vi "reward_behavior_michelle_visjitter_conswinAdapt_enticefx_TSLog_VF_fortraining_lightdetection2.vi"() -> ()   [LabVIEW 2019]
doc: "The myRIO Project template acquires acceleration data from the onboard accelerometer and displays the changes of acceleration values in a waveform chart."
uses:
  <vilib>/Analysis/Matrix/Datatypes/RealMatrix.ctl
  <vilib>/myRIO/Instrument Drivers/Onboard IO/DIO/typedefs/DIO Reference.ctl
  <vilib>/myRIO/Common/Instrument Driver Framework/Utilities/typedefs/myRIO Generic Hardware Reference.ctl
  <vilib>/myRIO/Common/Instrument Driver Framework/Utilities/typedefs/Hardware Version Enum.ctl
  <vilib>/myRIO/Common/Instrument Driver Framework/Utilities/typedefs/myRIO v1.0 Reference.ctl
  <vilib>/myRIO/Common/Instrument Driver Framework/Utilities/typedefs/Generic FPGA Reference.ctl
  <vilib>/myRIO/Common/Instrument Driver Framework/myRIO v1.0/DIO/typedefs/DIO Channels List.ctl
  <vilib>/myRIO/Common/Instrument Driver Framework/myRIO v1.0/DIO/typedefs/DIO Channels Enum.ctl
  <vilib>/userdefined/High Color/nirio_resource_hc.ctl
  <vilib>/myRIO/Common/Instrument Driver Framework/myRIO v1.0/Encoder/typedefs/Encoder Signal Mode.ctl
  <vilib>/myRIO/Instrument Drivers/Onboard IO/Encoder/typedefs/Encoder Reference.ctl
  <vilib>/myRIO/Common/Instrument Driver Framework/myRIO v1.0/Encoder/typedefs/Encoder Channels Enum.ctl
  <vilib>/myRIO/Common/Instrument Driver Framework/myRIO v1.0/Encoder/typedefs/Encoder Configuration v1.0.ctl
  <vilib>/myRIO/Instrument Drivers/Onboard IO/AI/typedefs/AI Reference.ctl
  <vilib>/myRIO/Common/Instrument Driver Framework/myRIO v1.0/AI/typedefs/AI Channels List.ctl
  <vilib>/myRIO/Common/Instrument Driver Framework/myRIO v1.0/AI/typedefs/AI Channels Enum.ctl
  <vilib>/myRIO/Common/Instrument Driver Framework/Utilities/typedefs/Analog Scaling Constants List.ctl
  <vilib>/myRIO/Common/Instrument Driver Framework/Utilities/typedefs/Analog Scaling Constants.ctl
  <vilib>/myRIO/Common/Instrument Driver Framework/Utilities/vis/Is FPGA Ref Available.vi
  <vilib>/myRIO/Common/Instrument Driver Framework/myRIO v1.0/DIO/vis/myRIO v1.1 Open DIO.vi
  <vilib>/myRIO/Instrument Drivers/Onboard IO/DIO/vis/Write.vi
  <vilib>/myRIO/Common/Instrument Driver Framework/myRIO v1.0/Encoder/vis/myRIO v1.1 Open Encoder.vi
  <vilib>/myRIO/Instrument Drivers/Onboard IO/Encoder/vis/Read.vi
  <vilib>/myRIO/Common/Instrument Driver Framework/myRIO v1.0/AI/vis/myRIO v1.1 Open AI.vi
  <vilib>/myRIO/Instrument Drivers/Onboard IO/AI/vis/Read.vi
  <vilib>/myRIO/Instrument Drivers/Onboard IO/DIO/vis/Read.vi
  <vilib>/myRIO/Common/Instrument Driver Framework/Utilities/vis/Validate Channels.vi
  <vilib>/myRIO/Common/Instrument Driver Framework/myRIO v1.0/DIO/vis/myRIO v1.0 Reserve DIO.vi
  <vilib>/myRIO/Common/Instrument Driver Framework/myRIO v1.0/Encoder/vis/myRIO v1.0 Reserve Encoder.vi
  <vilib>/myRIO/Common/Instrument Driver Framework/myRIO v1.0/AI/vis/myRIO v1.0 Reserve AI.vi
  <vilib>/myRIO/Common/Instrument Driver Framework/myRIO v1.0/Resource Manager/vis/myRIO v1.0 Reserve Channel List.vi
  <vilib>/myRIO/Common/Instrument Driver Framework/myRIO v1.0/DIO/vis/myRIO v1.0 Build MUX Configuration DIO.vi
  <vilib>/myRIO/Common/Instrument Driver Framework/myRIO v1.0/Encoder/vis/myRIO v1.0 Build MUX Configuration Encoder.vi
  <vilib>/myRIO/Common/Instrument Driver Framework/myRIO v1.0/AI/vis/myRIO v1.0 Build MUX Configuration AI.vi
  <vilib>/myRIO/Common/Instrument Driver Framework/myRIO v1.0/Resource Manager/vis/myRIO v1.0 Reserve Channel.vi
  <vilib>/myRIO/Common/Instrument Driver Framework/myRIO v1.0/Resource Manager/vis/myRIO v1.0 Unreserve Channel.vi
  <vilib>/myRIO/Common/Instrument Driver Framework/myRIO v1.0/Resource Manager/vis/myRIO v1.0 Create Configuration List.vi
  <vilib>/myRIO/Common/Instrument Driver Framework/myRIO v1.0/Resource Manager/vis/myRIO v1.0 Build Mutex Name.vi
  <vilib>/Utility/VariantDataType/GetNumericInfo.vi
  <vilib>/Utility/error.llb/Error Cluster From Error Code.vi
  <vilib>/myRIO/Common/Instrument Driver Framework/myRIO v1.0/myRIO v1.1 Open.vi
  <vilib>/myRIO/Common/Instrument Driver Framework/Utilities/vis/IO Manager.vi
  <vilib>/myRIO/Common/Instrument Driver Framework/Utilities/vis/Configuration Manager.vi
  <vilib>/myRIO/Common/Instrument Driver Framework/myRIO v1.0/Resource Manager/vis/myRIO v1.0 Configure IO.vi
  <vilib>/myRIO/Common/Instrument Driver Framework/myRIO v1.0/myRIO v1.0 Close.vi
  <vilib>/myRIO/Common/Instrument Driver Framework/myRIO v1.0/Encoder/vis/myRIO v1.0 Configure Encoder.vi
  <vilib>/myRIO/Common/Instrument Driver Framework/myRIO v1.0/Encoder/vis/myRIO v1.0 Read Encoder.vi
  <vilib>/myRIO/Common/Instrument Driver Framework/myRIO v1.0/DIO/vis/myRIO v1.0 Write DIO.vi
  <vilib>/myRIO/Common/Instrument Driver Framework/myRIO v1.0/DIO/vis/myRIO v1.0 Read DIO.vi
  <vilib>/myRIO/Common/Instrument Driver Framework/myRIO v1.0/AI/vis/myRIO v1.0 Get Scaling Constants AI.vi
  <vilib>/myRIO/Common/Instrument Driver Framework/myRIO v1.0/AI/vis/myRIO v1.0 Read AI.vi
  <vilib>/myRIO/Express VI/Onboard IO/Encoder/Encoder Express VI.xnode
  <vilib>/myRIO/Instrument Drivers/Onboard IO/Encoder/vis/myRIO Encoder Open.xnode
  <vilib>/myRIO/Common/Instrument Driver Framework/myRIO v1.0/Encoder/typedefs/Encoder Count Direction Enum.ctl
  <vilib>/myRIO/Express VI/Onboard IO/DO/DO Express VI.xnode
  <vilib>/myRIO/Instrument Drivers/Onboard IO/DIO/vis/myRIO DIO Open.xnode
  <vilib>/myRIO/Express VI/Onboard IO/DI/DI Express VI.xnode
  <vilib>/myRIO/Express VI/Onboard IO/AI/AI Express VI.xnode
  <vilib>/myRIO/Instrument Drivers/Onboard IO/AI/vis/myRIO AI Open.xnode
  <vilib>/myRIO/Instrument Drivers/Onboard IO/Encoder/Encoder.lvlib
  <vilib>/myRIO/Instrument Drivers/Onboard IO/DIO/DIO.lvlib
  <vilib>/myRIO/Instrument Drivers/Onboard IO/AI/AI.lvlib
  <vilib>/Analysis/Matrix/NI_Matrix.lvlib
panel:
  out "LightDeriv":dbl
  out "LightOn":bool=TRUE
  out "Light":dbl
  out "Lightplot":dbl[](graph)
  out "LightArray":dbl[](array[numeric])
  out "AutoEnticeLimit":i32=1000
  out "GetVidFrame":i32
  out "VidTS":dbl[][](array[numeric])
  out "VidFrameClock":i32
  out "EntTS":dbl[][](array[numeric])
  out "TimeLag":dbl
  out "Lag2":dbl
  out "TestTime":dbl
  out "RewTS":dbl[][](array[numeric])
  out "ConsTS":dbl[][](array[numeric])
  out "LickTS":dbl[][](array[numeric])
  out "ContrastChoice":dbl
  out "Its":i32
  out "BurstCriteria":dbl
  out "LickBurst 2":bool
  out "LickBurst":bool
  out "Enticements":i32
  in  "Entice":bool
  out "Misses":i32
  out "GoAhead":bool
  out "TimeOutDuration":i32
  out "ActiveTime":dbl
  out "ConsumptionGo":bool=TRUE
  out "Consumption_Period":i32
  out "Watch_Display":bool=TRUE
  in  "Give reward":bool
  out "Timings":dbl[](array[numeric])
  out "ISI":dbl
  out "ISI start time":dbl
  out "Time_out":bool=TRUE
  out "Time since lick":dbl
  out "Time of last lick":dbl
  out "Rewarded trials":dbl[](array[numeric])
  out "Rewards":u16
  out "Active Trial":bool
  out "Array temp2":T1
  out "Stimuli Loaded":bool
  out "Stim_ID":dbl[](array[numeric])
  out "Reward_mat":dbl[](array[numeric])
  out "Reward":bool=TRUE
  out "Frame clock":i32
  out "Licks":u32
  out "Lick":bool
  out "Time":dbl
  out "Stop":bool
  in  "Frames to collect":u32
  out "Overflow?":bool
  out "Counter Value":i32
  out "Velocity":dbl
  out "Velocity Plot":dbl[](graph)
  out "Velocity array":dbl[](array[numeric])
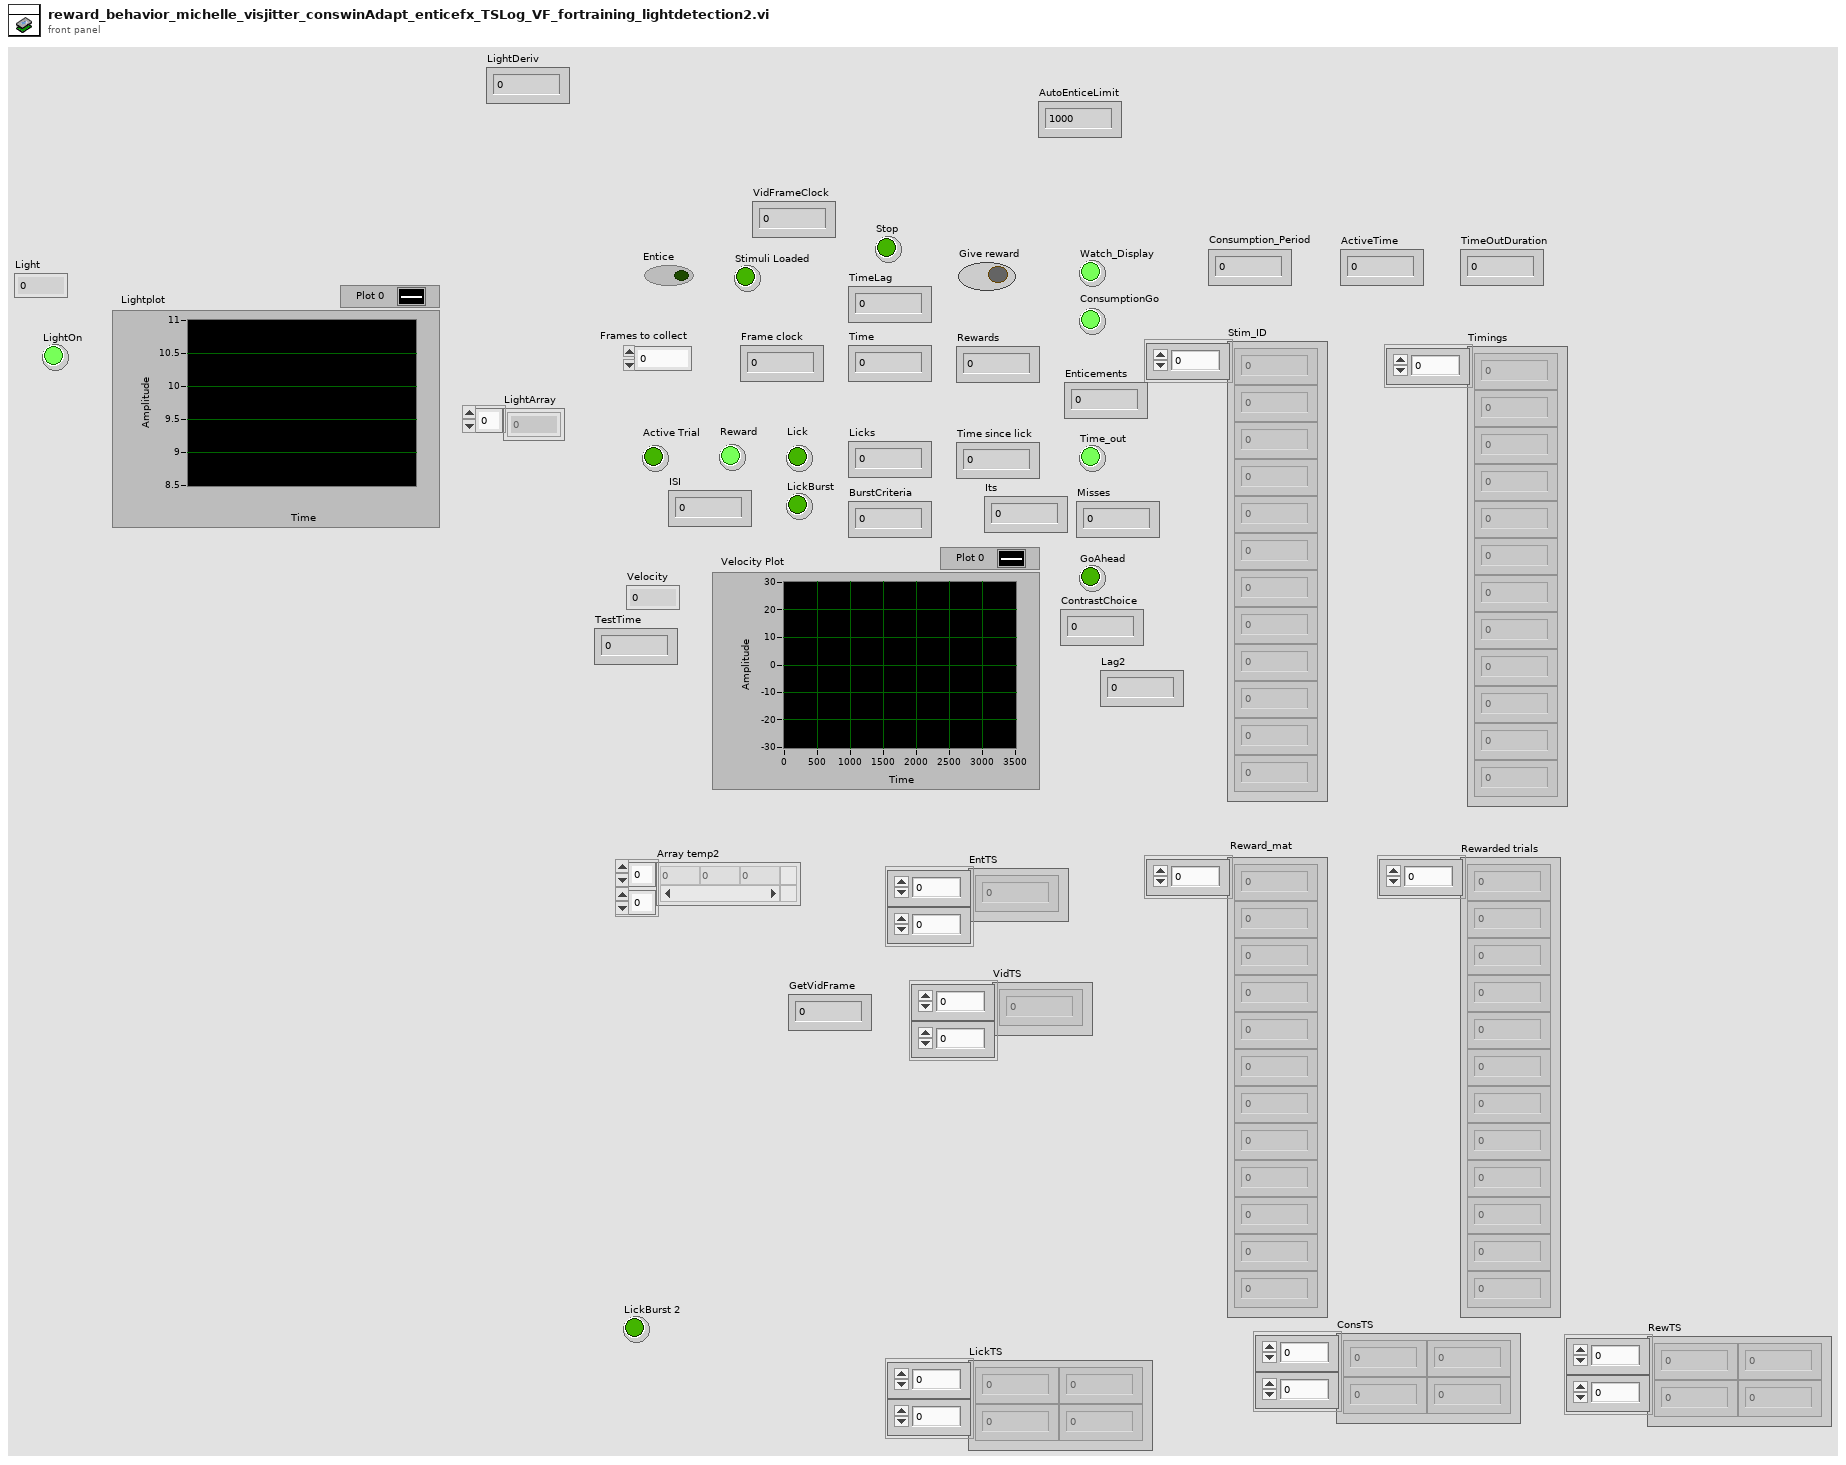
[diagram p1: front panel]
types:
  T1 = typedef "NI_Matrix.lvlib/RealMatrix.ctl" = dbl[][]
  T2 = typedef "DIO.lvlib/DIO Reference.ctl" = cluster{"myRIO Reference":T3, "DIO Channels List":T7}
  T3 = typedef "myRIO Generic Hardware Reference.ctl" = cluster{"myRIO Model":T4, "myRIO Hardware Reference":T5}
  T4 = typedef "Hardware Version Enum.ctl" = enum16{"Unknown", "myRIO-1900", "myRIO-1950", "roboRIO", "NI ELVIS RIO CM", "ELVIS III"}
  T5 = typedef "myRIO v1.0 Reference.ctl" = cluster{"Generic FPGA Reference":T6, "Allow multiple opens":bool}
  T6 = typedef "Generic FPGA Reference.ctl" = refnum<k20>
  T7 = typedef "DIO Channels List.ctl" = T8[]
  T8 = typedef "DIO Channels Enum.ctl" = enum16{"Not Connected", "C/DIO0", "C/DIO1", "C/DIO2", "C/DIO3", "C/DIO4", "C/DIO5", "C/DIO6", "C/DIO7", "A/DIO0", "A/DIO1", "A/DIO2", "A/DIO3", "A/DIO4", "A/DIO5", "A/DIO6", "A/DIO7", "A/DIO8", "A/DIO9", "A/DIO10", "A/DIO11", "A/DIO12", "A/DIO13", "A/DIO14", "A/DIO15", "A/DIO16", "A/DIO17", "A/DIO18", "A/DIO19", "B/DIO0", "B/DIO1", "B/DIO2", "B/DIO3", "B/DIO4", "B/DIO5", "B/DIO6", "B/DIO7", "B/DIO8", "B/DIO9", "B/DIO10", "B/DIO11", "B/DIO12", "B/DIO13", "B/DIO14", "B/DIO15", "B/DIO16", "B/DIO17", "B/DIO18", "B/DIO19", "LED0", "LED1", "LED2", "LED3", "Button0", "DIO/DIO0", "DIO/DIO1", "DIO/DIO2", "DIO/DIO3", "DIO/DIO4", "DIO/DIO5", "DIO/DIO6", "DIO/DIO7", "DIO/DIO8", "DIO/DIO9", "SPI/CS0", "SPI/CS1", "SPI/CS2", "SPI/CS3", "LED RADIO (Green)", "LED RADIO (Red)", "LED COMM (Green)", "LED COMM (Red)", "LED MODE (Green)", "LED MODE (Red)"}
  T9 = typedef "nirio_resource_hc.ctl" = tag
  T10 = typedef "Encoder.lvlib/Encoder Reference.ctl" = cluster{"myRIO Reference":T3, "Encoder Channels Enum":T11}
  T11 = typedef "Encoder Channels Enum.ctl" = enum16{"Not Connected", "C/ENC0", "C/ENC1", "A/ENC", "A/ENC0", "A/ENC1", "A/ENC2", "A/ENC3", "A/ENC4", "A/ENC5", "A/ENC6", "A/ENC7", "A/ENC8", "A/ENC9", "B/ENC", "B/ENC0", "B/ENC1", "B/ENC2", "B/ENC3", "B/ENC4", "B/ENC5", "B/ENC6", "B/ENC7", "B/ENC8", "B/ENC9", "DIO/ENC0", "DIO/ENC1", "DIO/ENC2", "DIO/ENC3", "DIO/ENC4"}
  T12 = typedef "Encoder Signal Mode.ctl" = enum16{"Quadrature phase signal", "Step and direction signal"}
  T13 = typedef "AI.lvlib/AI Reference.ctl" = cluster{"myRIO Reference":T3, "AI Channels List":T14, "AI Scaling Constants List":T16}
  T14 = typedef "AI Channels List.ctl" = T15[]
  T15 = typedef "AI Channels Enum.ctl" = enum16{"Not Connected", "AudioIn/Left", "AudioIn/Right", "C/AI0", "C/AI1", "A/AI0", "A/AI1", "A/AI2", "A/AI3", "A/AI4", "A/AI5", "A/AI6", "A/AI7", "B/AI0", "B/AI1", "B/AI2", "B/AI3", "B/AI4", "B/AI5", "B/AI6", "B/AI7", "AI/AI0", "AI/AI1", "AI/AI2", "AI/AI3", "A/AI0 (DIFF)", "A/AI1 (DIFF)", "A/AI2 (DIFF)", "A/AI3 (DIFF)", "B/AI0 (DIFF)", "B/AI1 (DIFF)", "B/AI2 (DIFF)", "B/AI3 (DIFF)"}
  T16 = typedef "Analog Scaling Constants List.ctl" = T17[]
  T17 = typedef "Analog Scaling Constants.ctl" = cluster{"LSB Weight (Volts)":dbl, "Offset (Volts)":dbl, "Signed?":bool}
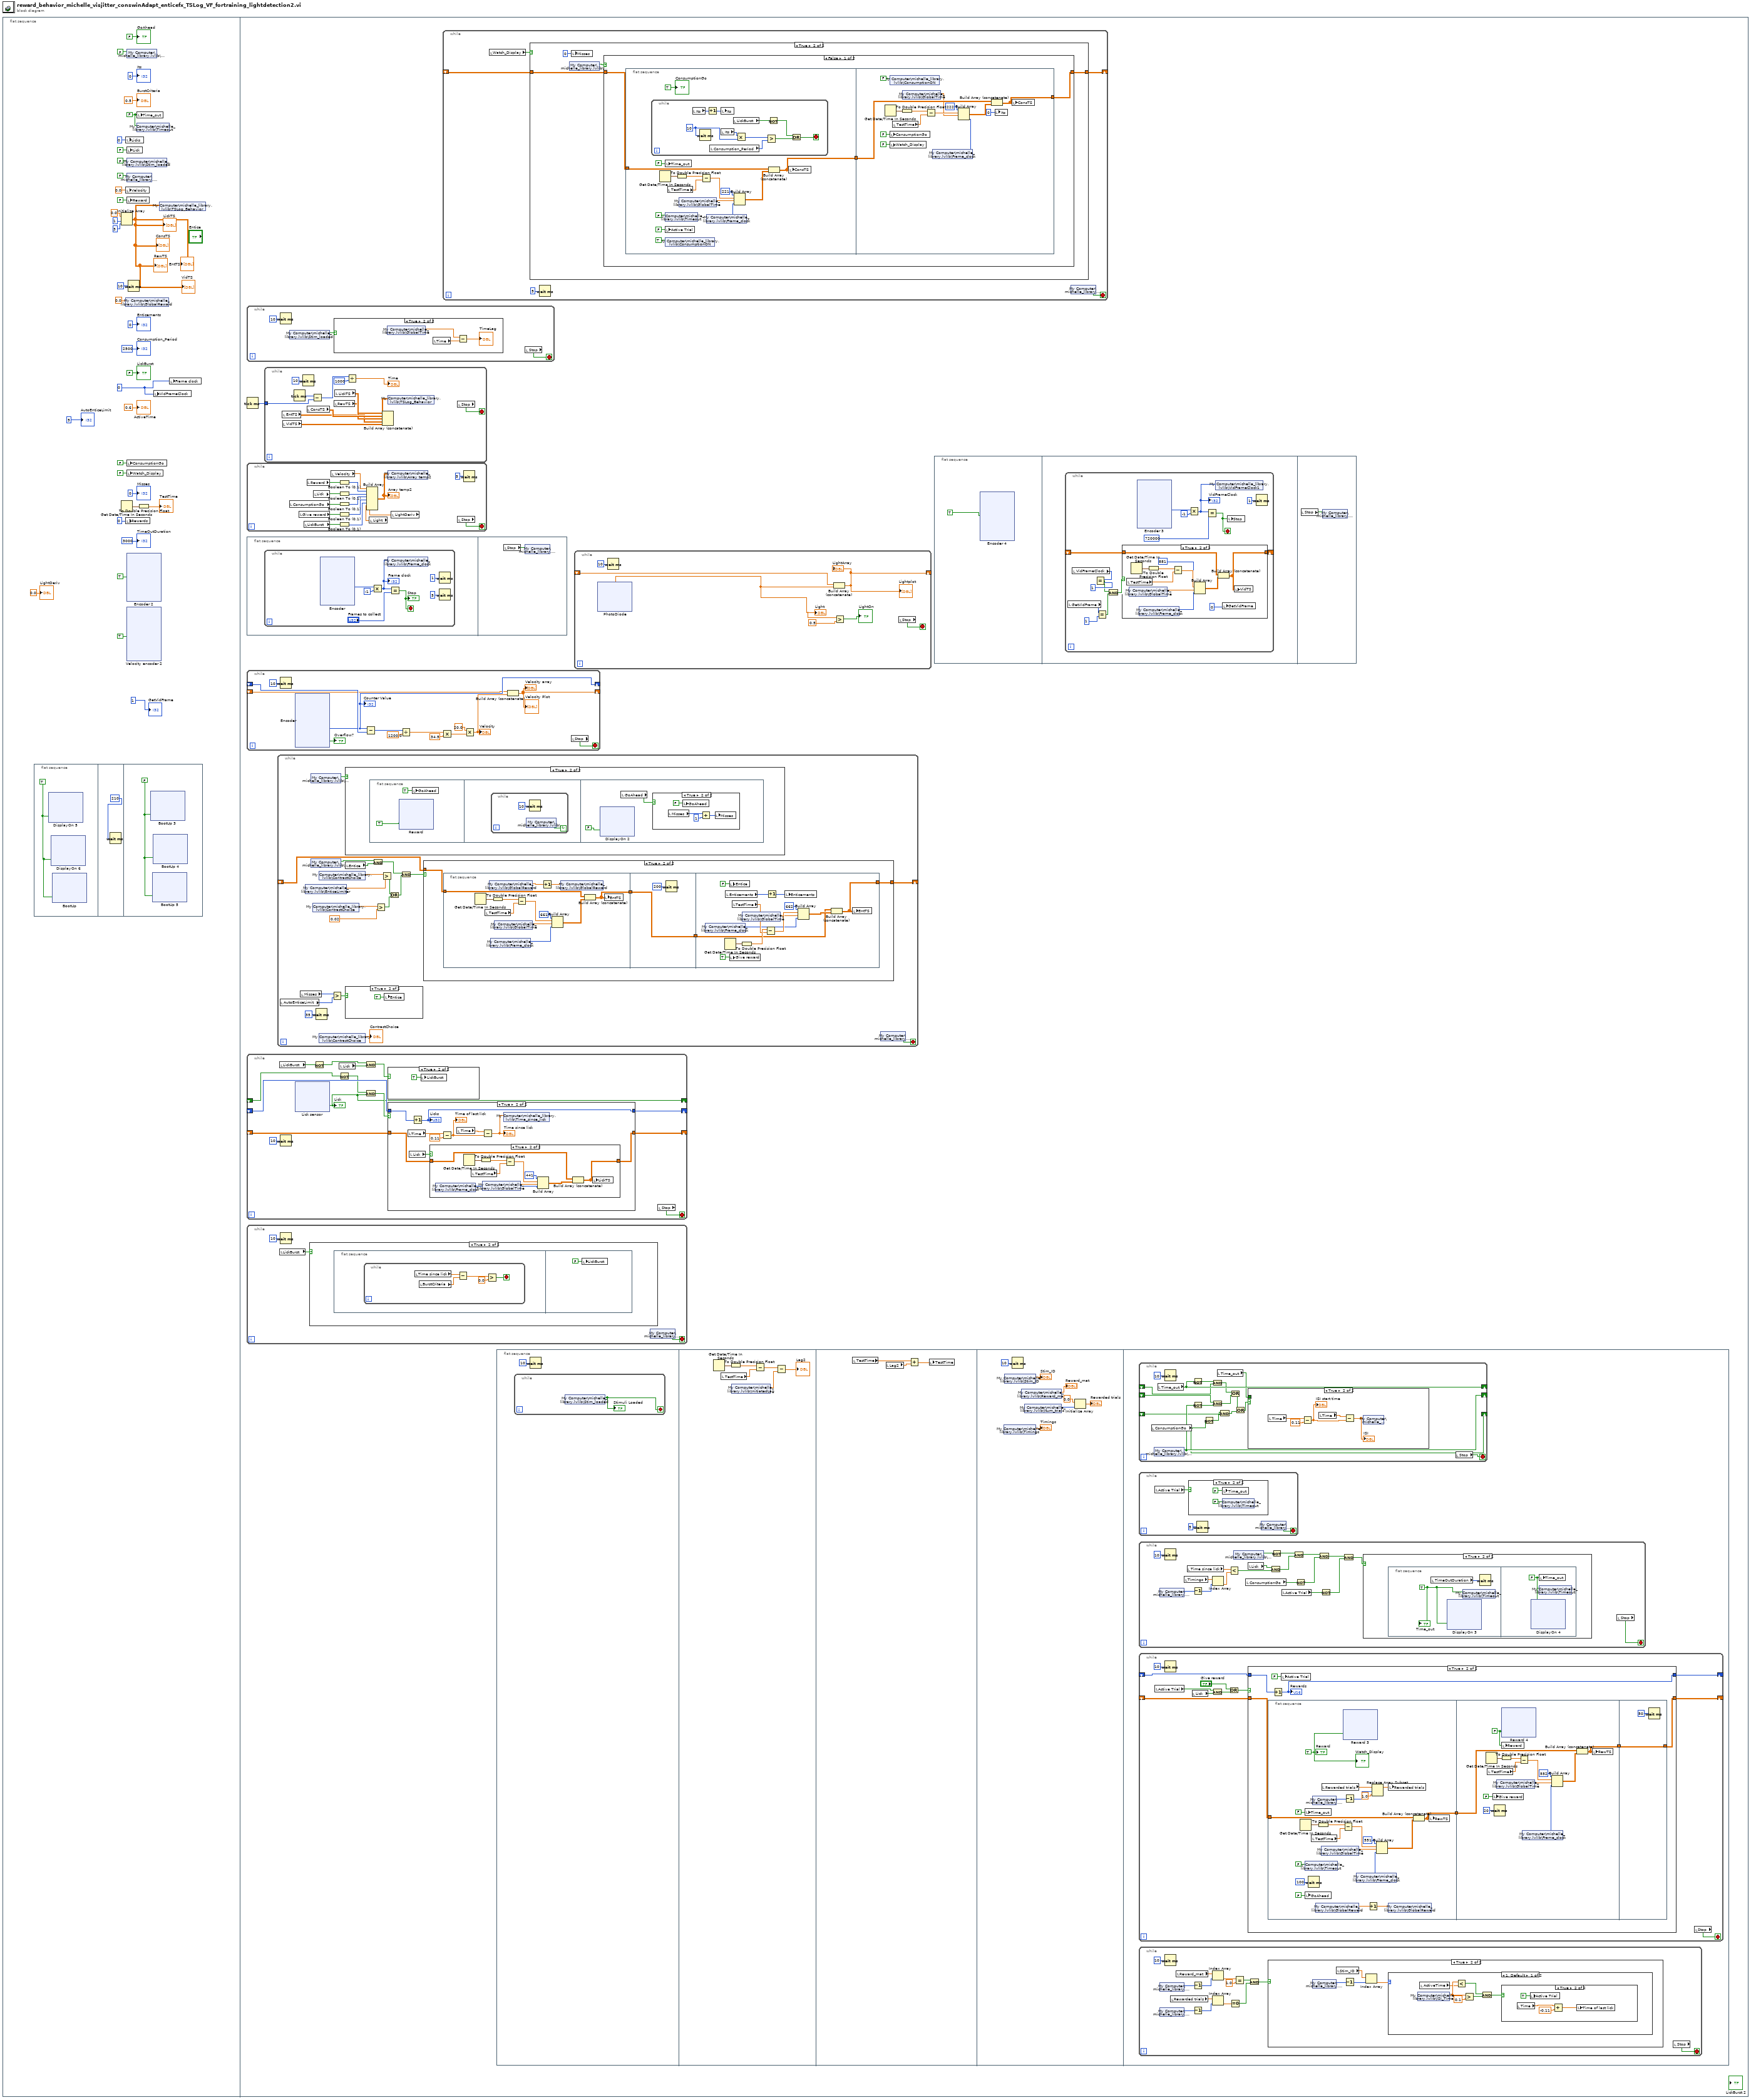
[diagram p0: block diagram]
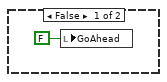
[diagram p7: hidden frame]
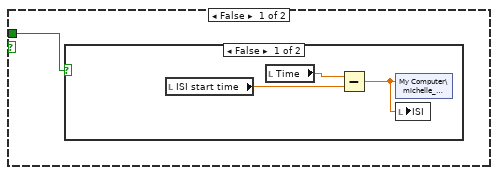
[diagram p13: hidden frame]
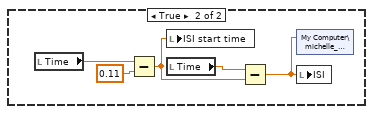
[diagram p14: hidden frame]
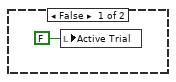
[diagram p15: hidden frame]
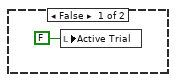
[diagram p16: hidden frame]
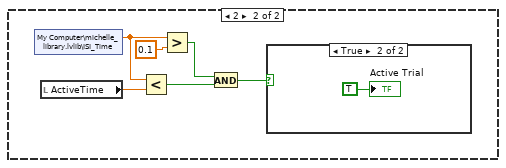
[diagram p17: hidden frame]
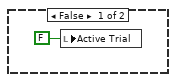
[diagram p18: hidden frame]
diagram:
  n1 = flat-sequence {
    frame #0 {
      w23 = FALSE ("Time_out")
      w5 = u32 0 ("Frames")
      n2 = flat-sequence {
        frame #0 {
          w35 = TRUE
          n3 = xnode "DisplayOn 5"("C/DIO2 (DIO2)"=w35) -> ()  [unwired: 1 in, 1 out]
          n4 = xnode "DisplayOn 6"("C/DIO1 (DIO1)"=w35) -> ()  [unwired: 1 in, 1 out]
          n5 = xnode "BootUp"("C/DIO3 (DIO3)"=w35) -> ()  [unwired: 1 in, 1 out]
        }
        frame #1 {
          n6 = Wait (ms)(milliseconds to wait=210) -> ()  [unwired: 1 out]
        }
        frame #2 {
          w142 = FALSE
          n7 = xnode "BootUp 3"("C/DIO2 (DIO2)"=w142) -> ()  [unwired: 1 in, 1 out]
          n8 = xnode "BootUp 5"("C/DIO3 (DIO3)"=w142) -> ()  [unwired: 1 in, 1 out]
          n9 = xnode "BootUp 4"("C/DIO1 (DIO1)"=w142) -> ()  [unwired: 1 in, 1 out]
        }
      }
      n10 = Get Date/Time In Seconds() -> (seconds since 1Jan1904=w7:timestamp)
      n11 = Initialize Array(0.0, 1, 3) -> (w4:dbl[][])
      "LickTS" <- w4
      "ConsTS" <- w4
      "RewTS" <- w4
      "EntTS" <- w4
      "VidTS" <- w4
      n12 = local write "Licks"(u32 0 ("Licks")) -> ()
      n13 = local write "Velocity"(0.0 ("Velocity")) -> ()
      n14 = shared-variable "My Computer\\michelle_library.lvlib\\GlobalReward"(0.0) -> ()  [unwired: 1 in, 1 out]
      n15 = local write "Rewards"(u16 0 ("Rewards")) -> ()
      n16 = shared-variable "My Computer\\michelle_library.lvlib\\Display"(FALSE ("Display")) -> ()  [unwired: 1 in, 1 out]
      n17 = local write "Lick"(FALSE ("Lick")) -> ()
      n18 = shared-variable "My Computer\\michelle_library.lvlib\\Stim_loaded"(FALSE ("Stim_loaded")) -> ()  [unwired: 1 in, 1 out]
      n19 = shared-variable "My Computer\\michelle_library.lvlib\\Stop"(FALSE ("Stop")) -> ()  [unwired: 1 in, 1 out]
      n20 = local write "Reward"(FALSE ("Give reward")) -> ()
      n21 = local write "ConsumptionGo"(FALSE ("ConsumptionGo")) -> ()
      n22 = local write "Watch_Display"(FALSE ("Watch_Display")) -> ()
      n23 = xnode "Encoder 2"("Reset Counter"=TRUE) -> ()  [unwired: 1 in, 4 out]
      n24 = xnode "Velocity encoder 2"("Reset Counter"=TRUE) -> ()  [unwired: 1 in, 4 out]
      n25 = Wait (ms)(milliseconds to wait=u32 10) -> ()  [unwired: 1 out]
      n26 = local write "Time_out"(w23) -> ()
      n27 = shared-variable "My Computer\\michelle_library.lvlib\\Timeout"(w23) -> ()  [unwired: 1 in, 1 out]
      n28 = To Double Precision Float(number=w7) -> (double precision float=→"TestTime":dbl)
      n29 = local write "VidFrameClock"(w5) -> ()
      n30 = shared-variable "My Computer\\michelle_library.lvlib\\TSLog_Behavior"(w4) -> ()  [unwired: 1 in, 1 out]
      n31 = local write "Frame clock"(w5) -> ()
      "Consumption_Period" <- 2500
      "ActiveTime" <- 0.6
      "TimeOutDuration" <- 3000
      "GoAhead" <- FALSE
      "Misses" <- 0
      "Enticements" <- 0
      "LickBurst" <- FALSE
      "BurstCriteria" <- 0.5
      "Its" <- 0
      "GetVidFrame" <- 1
      "AutoEnticeLimit" <- 5
      "LightDeriv" <- 0.0
    }
    frame #1 {
      n32 = while {
        stop <- w507 stop-if-true
        n33 = Wait (ms)(milliseconds to wait=u32 10) -> ()  [unwired: 1 out]
        n34 = shared-variable "My Computer\\michelle_library.lvlib\\Stim_loaded"() -> (w508:bool)  [unwired: 1 in, 1 out]
        n35 = case shown="True" w508 {
          frame False {
          }
          frame True {
            n36 = shared-variable "My Computer\\michelle_library.lvlib\\GlobalTime"() -> (w509:dbl)  [unwired: 1 in, 1 out]
            n37 = local read "Time"() -> (w510:dbl)
            n38 = Subtract(x=w509, y=w510) -> (x-y=→"TimeLag":dbl)
          }
        }
        n39 = local read "Stop"() -> (w507:bool)
      }
      n40 = Tick Count (ms)() -> (millisecond timer value=w340:u32)
      n41 = while {
        stop <- w718 stop-if-true
        n42 = local read "ConsumptionGo"() -> (w716:bool)
        n43 = local read "Give reward"() -> (w715:bool)
        n44 = local read "LickBurst"() -> (w712:bool)
        n45 = local read "Reward"() -> (w723:bool)
        n46 = local read "Lick"() -> (w724:bool)
        n47 = local read "Velocity"() -> (w722:dbl)
        n48 = Boolean To (0,1)(Boolean=w723) -> (0, 1=w721:i16)
        n49 = Boolean To (0,1)(Boolean=w724) -> (0, 1=w720:i16)
        n50 = Boolean To (0,1)(Boolean=w716) -> (0, 1=w714:i16)
        n51 = Boolean To (0,1)(Boolean=w715) -> (0, 1=w713:i16)
        n52 = Boolean To (0,1)(Boolean=w712) -> (0, 1=w711:i16)
        n53 = local read "Light"() -> (w710:dbl)
        n54 = local read "LightDeriv"() -> (w709:dbl)
        n55 = Build Array(w722, w721, w720, w714, w713, w711, w710, w709) -> (w717:T1)
        "Array temp2" <- w717
        n56 = shared-variable "My Computer\\michelle_library.lvlib\\Array temp2"(w717) -> ()  [unwired: 1 in, 1 out]
        n57 = local read "Stop"() -> (w718:bool)
        n58 = Wait (ms)(milliseconds to wait=u32 5) -> ()  [unwired: 1 out]
      }
      n59 = flat-sequence {
        frame #0 {
          n60 = while {
            stop <- w1037 stop-if-true
            n61 = xnode "Encoder"() -> ("Counter Value"=w1041:i32)  [unwired: 2 in, 3 out]
            n62 = Multiply(x=w1041, y=-1) -> (x*y=w1036:i32)
            "Frame clock" <- w1036
            n63 = shared-variable "My Computer\\michelle_library.lvlib\\Frame_clock"(w1036) -> ()  [unwired: 1 in, 1 out]
            n64 = Equal?(x=w1036, y="Frames to collect") -> (x = y?=w1037:bool)
            "Stop" <- w1037
            n65 = Wait (ms)(milliseconds to wait=u32 1) -> ()  [unwired: 1 out]
            n66 = Wait (ms)(milliseconds to wait=u32 5) -> ()  [unwired: 1 out]
          }
        }
        frame #1 {
          n67 = local read "Stop"() -> (w1089:bool)
          n68 = shared-variable "My Computer\\michelle_library.lvlib\\Stop"(w1089) -> ()  [unwired: 1 in, 1 out]
        }
      }
      n69 = while {
        shift-right: [w1176] -> _
        shift-left: _ -> [w1177]
        shift-right: [w1168] -> _
        shift-left: _ -> [w1167]
        stop <- w1166 stop-if-true
        n70 = Wait (ms)(milliseconds to wait=u32 10) -> ()  [unwired: 1 out]
        n71 = xnode "Encoder"() -> ("Counter Value"=w1176:i32, "Overflow?"=→"Overflow?":bool)  [unwired: 2 in, 2 out]
        "Counter Value" <- w1176
        n72 = Subtract(x=w1176, y=w1177) -> (x-y=w1169:i32)
        n73 = Divide(x=w1169, y=1200.0 ("600")) -> (x/y=w1174:dbl)
        n74 = Multiply(x=w1174, y=34.5) -> (x*y=w1172:dbl)
        n75 = Multiply(x=20.0, y=w1172) -> (x*y=w1170:dbl)
        "Velocity" <- w1170
        n76 = Build Array (concatenate)(w1167, w1170) -> (w1168:dbl[])
        "Velocity Plot" <- w1168
        "Velocity array" <- w1168
        n77 = local read "Stop"() -> (w1166:bool)
      }
      n78 = while {
        shift-right: [w1102] -> _
        shift-left: _ -> [w1101]
        shift-right: [w1096] -> _
        shift-left: _ -> [w1099]
        shift-right: [w1090] -> _
        shift-left: _ -> [w1091]
        stop <- w1100 stop-if-true
        n79 = local read "LickBurst"() -> (w1093:bool)
        n80 = Wait (ms)(milliseconds to wait=u32 10) -> ()  [unwired: 1 out]
        n81 = xnode "Lick sensor"() -> ("C/DIO1 (DIO1)"=w1096:bool)  [unwired: 1 in, 1 out]
        "Lick" <- w1096
        n82 = Not(x=w1093) -> (.not. x?=w1092:bool)
        n83 = Not(x=w1099) -> (.not. x?=w1098:bool)
        n84 = local read "Lick"() -> (w1094:bool)
        n85 = And(x=w1092, y=w1094) -> (x .and. y?=w1095:bool)
        n86 = And(x=w1098, y=w1096) -> (x .and. y?=w1097:bool)
        n87 = case shown="True" w1095 {
          frame False {
          }
          frame True {
            n88 = local write "LickBurst"(TRUE) -> ()
          }
        }
        n89 = case shown="True" w1097 {
          tunnel: [w1109 w1119] -> w1102
          tunnel: w1101 -> [w1109 w1118]
          tunnel: w1091 -> [w1105 w1110]
          tunnel: [w1105 w1112] -> w1090
          frame False {
            n90 = local read "Time of last lick"() -> (w1107:dbl)
            n91 = local read "Time"() -> (w1108:dbl)
            n92 = Subtract(x=w1108, y=w1107) -> (x-y=w1106:dbl)
            n93 = shared-variable "My Computer\\michelle_library.lvlib\\Time_since_lick"(w1106) -> ()  [unwired: 1 in, 1 out]
            n94 = local write "Time since lick"(w1106) -> ()
          }
          frame True {
            n95 = local read "Time"() -> (w1115:dbl)
            n96 = local read "Lick"() -> (w1111:bool)
            n97 = Increment(x=w1118) -> (x+1=w1119:u32)
            "Licks" <- w1119
            n98 = case shown="True" w1111 {
              tunnel: w1110 -> [w1120 w1126]
              tunnel: [w1120 w1125] -> w1112
              frame False {
              }
              frame True {
                n99 = shared-variable "My Computer\\michelle_library.lvlib\\Frame_clock"() -> (w1121:u32)  [unwired: 1 in, 1 out]
                n100 = Get Date/Time In Seconds() -> (seconds since 1Jan1904=w1128:timestamp)
                n101 = local read "TestTime"() -> (w1123:dbl)
                n102 = To Double Precision Float(number=w1128) -> (double precision float=w1124:dbl)
                n103 = shared-variable "My Computer\\michelle_library.lvlib\\GlobalTime"() -> (w1122:dbl)  [unwired: 1 in, 1 out]
                n104 = Subtract(x=w1124, y=w1123) -> (x-y=w1129:dbl)
                n105 = Build Array(441, w1129, w1122, w1121) -> (w1130:T1)
                n106 = Build Array (concatenate) ("Build Matrix")(w1126, w1130) -> (w1125:T1)
                n107 = local write "LickTS"(w1125) -> ()
              }
            }
            n108 = Subtract(x=w1115, y=0.11) -> (x-y=w1113:dbl)
            "Time of last lick" <- w1113
            n109 = local read "Time"() -> (w1117:dbl)
            n110 = Subtract(x=w1117, y=w1113) -> (x-y=w1116:dbl)
            "Time since lick" <- w1116
            n111 = shared-variable "My Computer\\michelle_library.lvlib\\Time_since_lick"(w1116) -> ()  [unwired: 1 in, 1 out]
          }
        }
        n112 = local read "Stop"() -> (w1100:bool)
      }
      n113 = while {
        stop <- w514 stop-if-true
        n114 = local read "LickBurst"() -> (w512:bool)
        n115 = Wait (ms)(milliseconds to wait=u32 10) -> ()  [unwired: 1 out]
        n116 = case shown="True" w512 {
          frame False {
          }
          frame True {
            n117 = flat-sequence {
              frame #0 {
                n118 = while {
                  stop <- w517 stop-if-true
                  n119 = local read "Time since lick"() -> (w518:dbl)
                  n120 = local read "BurstCriteria"() -> (w519:dbl)
                  n121 = Subtract(x=w518, y=w519) -> (x-y=w515:dbl)
                  n122 = Greater?(x=w515, y=0.0) -> (0:w517:bool)
                }
              }
              frame #1 {
                n123 = local write "LickBurst"(FALSE) -> ()
              }
            }
          }
        }
        n124 = shared-variable "My Computer\\michelle_library.lvlib\\Stop"() -> (w514:bool)  [unwired: 1 in, 1 out]
      }
      n125 = while {
        tunnel: w340 -> [w1237]
        stop <- w1235 stop-if-true
        n126 = local read "EntTS"() -> (w1227:dbl[][])
        n127 = local read "VidTS"() -> (w1226:dbl[][])
        n128 = Tick Count (ms)() -> (millisecond timer value=w1238:u32)
        n129 = Wait (ms)(milliseconds to wait=u32 10) -> ()  [unwired: 1 out]
        n130 = local read "ConsTS"() -> (w1230:dbl[][])
        n131 = Subtract(x=w1238, y=w1237) -> (x-y=w1234:u32)
        n132 = local read "RewTS"() -> (w1229:dbl[][])
        n133 = local read "LickTS"() -> (w1231:dbl[][])
        n134 = Divide(x=w1234, y=u32 1000) -> (x/y=→"Time":dbl)
        n135 = Build Array (concatenate) ("Build Matrix")(w1231, w1230, w1229, w1227, w1226) -> (w1228:T1)
        n136 = shared-variable "My Computer\\michelle_library.lvlib\\TSLog_Behavior"(w1228) -> ()  [unwired: 1 in, 1 out]
        n137 = local read "Stop"() -> (w1235:bool)
      }
      n138 = while {
        shift-right: [w529] -> _
        shift-left: _ -> [w530]
        stop <- w540 stop-if-true
        n139 = local read "AutoEnticeLimit"() -> (w521:i32)
        n140 = local read "Misses"() -> (w522:i32)
        n141 = shared-variable "My Computer\\michelle_library.lvlib\\EnticeLimiter"() -> (w528:dbl)  [unwired: 1 in, 1 out]
        n142 = shared-variable "My Computer\\michelle_library.lvlib\\Display"() -> (w539:bool)  [unwired: 1 in, 1 out]
        n143 = shared-variable "My Computer\\michelle_library.lvlib\\Display"() -> (w537:bool)  [unwired: 1 in, 1 out]
        n144 = shared-variable "My Computer\\michelle_library.lvlib\\ContrastChoice"() -> (w524:dbl)  [unwired: 1 in, 1 out]
        n145 = Wait (ms)(milliseconds to wait=35) -> ()  [unwired: 1 out]
        n146 = shared-variable "My Computer\\michelle_library.lvlib\\ContrastChoice"() -> (w533:dbl)  [unwired: 1 in, 1 out]
        n147 = shared-variable "My Computer\\michelle_library.lvlib\\ContrastChoice"() -> (→"ContrastChoice":dbl)  [unwired: 1 in, 1 out]
        n148 = Greater?(x=w522, y=w521) -> (0:w538:bool)
        n149 = case shown="True" w539 {
          frame False {
            n150 = local write "GoAhead"(FALSE) -> ()
          }
          frame True {
            n151 = flat-sequence {
              frame #0 {
                n152 = xnode "Reward"("C/DIO2 (DIO2)"=TRUE) -> ()  [unwired: 1 in, 1 out]
                n153 = local write "GoAhead"(TRUE) -> ()
              }
              frame #1 {
                n154 = while {
                  stop <- w614 continue-if-true
                  n155 = shared-variable "My Computer\\michelle_library.lvlib\\Display"() -> (w614:bool)  [unwired: 1 in, 1 out]
                  n156 = Wait (ms)(milliseconds to wait=10) -> ()  [unwired: 1 out]
                }
              }
              frame #2 {
                n157 = xnode "DisplayOn 2"("C/DIO2 (DIO2)"=FALSE) -> ()  [unwired: 1 in, 1 out]
                n158 = local read "GoAhead"() -> (w616:bool)
                n159 = case shown="True" w616 {
                  frame False {
                  }
                  frame True {
                    n160 = local read "Misses"() -> (w655:i32)
                    n161 = local write "GoAhead"(FALSE) -> ()
                    n162 = Add(x=w655, y=1) -> (x+y=w653:i32)
                    n163 = local write "Misses"(w653) -> ()
                  }
                }
              }
            }
          }
        }
        n164 = local read "Entice"() -> (w536:bool)
        n165 = case shown="True" w538 {
          frame False {
          }
          frame True {
            n166 = local write "Entice"(TRUE) -> ()
          }
        }
        n167 = And(x=w537, y=w536) -> (x .and. y?=w534:bool)
        n168 = Greater?(x=w524, y=0.02) -> (0:w525:bool)
        n169 = Greater?(x=w533, y=w528) -> (0:w526:bool)
        n170 = Or(x=w526, y=w525) -> (x .or. y?=w527:bool)
        n171 = And(x=w534, y=w527) -> (x .and. y?=w532:bool)
        n172 = case shown="True" w532 {
          tunnel: w530 -> [w541 w545]
          tunnel: [w541 w542] -> w529
          frame False {
          }
          frame True {
            n173 = flat-sequence {
              tunnel: w545 -> [w548]
              tunnel: [w547] -> w544
              tunnel: w544 -> [w558]
              tunnel: [w558] -> w543
              tunnel: w543 -> [w562]
              tunnel: [w561] -> w542
              frame #0 {
                n174 = Get Date/Time In Seconds() -> (seconds since 1Jan1904=w555:timestamp)
                n175 = local read "TestTime"() -> (w550:dbl)
                n176 = shared-variable "My Computer\\michelle_library.lvlib\\GlobalReward"() -> (w557:dbl)  [unwired: 1 in, 1 out]
                n177 = shared-variable "My Computer\\michelle_library.lvlib\\Frame_clock"() -> (w546:u32)  [unwired: 1 in, 1 out]
                n178 = To Double Precision Float(number=w555) -> (double precision float=w554:dbl)
                n179 = shared-variable "My Computer\\michelle_library.lvlib\\GlobalTime"() -> (w549:dbl)  [unwired: 1 in, 1 out]
                n180 = Subtract(x=w554, y=w550) -> (x-y=w553:dbl)
                n181 = Increment(x=w557) -> (x+1=w556:dbl)
                n182 = Build Array(661, w553, w549, w546) -> (w552:T1)
                n183 = shared-variable "My Computer\\michelle_library.lvlib\\GlobalReward"(w556) -> ()  [unwired: 1 in, 1 out]
                n184 = Build Array (concatenate) ("Build Matrix")(w548, w552) -> (w547:T1)
                n185 = local write "EntTS"(w547) -> ()
              }
              frame #1 {
                n186 = Wait (ms)(milliseconds to wait=200) -> ()  [unwired: 1 out]
              }
              frame #2 {
                n187 = shared-variable "My Computer\\michelle_library.lvlib\\Frame_clock"() -> (w560:u32)  [unwired: 1 in, 1 out]
                n188 = Get Date/Time In Seconds() -> (seconds since 1Jan1904=w569:timestamp)
                n189 = local read "Enticements"() -> (w571:i32)
                n190 = local write "Entice"(FALSE) -> ()
                n191 = local write "Give reward"(TRUE) -> ()
                n192 = local read "TestTime"() -> (w563:dbl)
                n193 = To Double Precision Float(number=w569) -> (double precision float=w568:dbl)
                n194 = shared-variable "My Computer\\michelle_library.lvlib\\GlobalTime"() -> (w564:dbl)  [unwired: 1 in, 1 out]
                n195 = Subtract(x=w568, y=w563) -> (x-y=w567:dbl)
                n196 = Increment(x=w571) -> (x+1=w570:i32)
                n197 = local write "Enticements"(w570) -> ()
                n198 = Build Array(662, w567, w564, w560) -> (w566:T1)
                n199 = Build Array (concatenate) ("Build Matrix")(w562, w566) -> (w561:T1)
                n200 = local write "EntTS"(w561) -> ()
              }
            }
          }
        }
        n201 = shared-variable "My Computer\\michelle_library.lvlib\\Stop"() -> (w540:bool)  [unwired: 1 in, 1 out]
      }
      n202 = while {
        shift-right: [w656] -> _
        shift-left: _ -> [w657]
        stop <- w660 stop-if-true
        n203 = local read "Watch_Display"() -> (w659:bool)
        n204 = case shown="True" w659 {
          tunnel: w657 -> [w661 w663]
          tunnel: [w661 w662] -> w656
          frame False {
          }
          frame True {
            n205 = shared-variable "My Computer\\michelle_library.lvlib\\Display"() -> (w665:bool)  [unwired: 1 in, 1 out]
            n206 = local write "Misses"(0) -> ()
            n207 = case shown="False" w665 {
              tunnel: w663 -> [w668 w708]
              tunnel: [w666 w708] -> w662
              frame False {
                n208 = flat-sequence {
                  tunnel: w668 -> [w672]
                  tunnel: [w671] -> w667
                  tunnel: w667 -> [w698]
                  tunnel: [w697] -> w666
                  frame #0 {
                    n209 = while {
                      stop <- w687 stop-if-true
                      w688 = 10
                      n210 = local read "Its"() -> (w692:i32)
                      n211 = Wait (ms)(milliseconds to wait=w688) -> ()  [unwired: 1 out]
                      n212 = Increment(x=w692) -> (x+1=w691:i32)
                      n213 = local read "Consumption_Period"() -> (w685:i32)
                      n214 = local write "Its"(w691) -> ()
                      n215 = local read "Its"() -> (w689:i32)
                      n216 = local read "LickBurst"() -> (w693:bool)
                      n217 = Multiply(x=w689, y=w688) -> (x*y=w686:i32)
                      n218 = Greater?(x=w686, y=w685) -> (0:w684:bool)
                      n219 = Not(x=w693) -> (.not. x?=w690:bool)
                      n220 = Or(x=w690, y=w684) -> (x .or. y?=w687:bool)
                    }
                    n221 = Get Date/Time In Seconds() -> (seconds since 1Jan1904=w677:timestamp)
                    n222 = local write "Time_out"(FALSE) -> ()
                    n223 = shared-variable "My Computer\\michelle_library.lvlib\\Timeout"(FALSE) -> ()  [unwired: 1 in, 1 out]
                    n224 = local write "Active Trial"(FALSE) -> ()
                    n225 = shared-variable "My Computer\\michelle_library.lvlib\\ConsumptionON"(TRUE) -> ()  [unwired: 1 in, 1 out]
                    n226 = local read "TestTime"() -> (w674:dbl)
                    n227 = To Double Precision Float(number=w677) -> (double precision float=w675:dbl)
                    n228 = shared-variable "My Computer\\michelle_library.lvlib\\GlobalTime"() -> (w670:dbl)  [unwired: 1 in, 1 out]
                    n229 = Subtract(x=w675, y=w674) -> (x-y=w678:dbl)
                    n230 = shared-variable "My Computer\\michelle_library.lvlib\\Frame_clock"() -> (w669:u32)  [unwired: 1 in, 1 out]
                    n231 = Build Array(221, w678, w670, w669) -> (w673:T1)
                    n232 = Build Array (concatenate) ("Build Matrix")(w672, w673) -> (w671:T1)
                    n233 = local write "ConsTS"(w671) -> ()
                    "ConsumptionGo" <- TRUE
                  }
                  frame #1 {
                    n234 = Get Date/Time In Seconds() -> (seconds since 1Jan1904=w702:timestamp)
                    n235 = shared-variable "My Computer\\michelle_library.lvlib\\ConsumptionON"(FALSE) -> ()  [unwired: 1 in, 1 out]
                    n236 = local write "ConsumptionGo"(FALSE ("ConsumptionGo")) -> ()
                    n237 = local write "Watch_Display"(FALSE ("Watch_Display")) -> ()
                    n238 = local read "TestTime"() -> (w699:dbl)
                    n239 = To Double Precision Float(number=w702) -> (double precision float=w700:dbl)
                    n240 = shared-variable "My Computer\\michelle_library.lvlib\\GlobalTime"() -> (w695:dbl)  [unwired: 1 in, 1 out]
                    n241 = Subtract(x=w700, y=w699) -> (x-y=w703:dbl)
                    n242 = shared-variable "My Computer\\michelle_library.lvlib\\Frame_clock"() -> (w694:u32)  [unwired: 1 in, 1 out]
                    n243 = Build Array(222, w703, w695, w694) -> (w696:T1)
                    n244 = Build Array (concatenate) ("Build Matrix")(w698, w696) -> (w697:T1)
                    n245 = local write "Its"(0) -> ()
                    n246 = local write "ConsTS"(w697) -> ()
                  }
                }
              }
              frame True {
              }
            }
          }
        }
        n247 = Wait (ms)(milliseconds to wait=u32 5) -> ()  [unwired: 1 out]
        n248 = shared-variable "My Computer\\michelle_library.lvlib\\Stop"() -> (w660:bool)  [unwired: 1 in, 1 out]
      }
      n249 = flat-sequence {
        frame #0 {
          n250 = while {
            stop <- w726 stop-if-true
            n251 = shared-variable "My Computer\\michelle_library.lvlib\\Stim_loaded"() -> (w726:bool)  [unwired: 1 in, 1 out]
            "Stimuli Loaded" <- w726
          }
          n252 = Wait (ms)(milliseconds to wait=u32 10) -> ()  [unwired: 1 out]
        }
        frame #1 {
          n253 = Get Date/Time In Seconds() -> (seconds since 1Jan1904=w732:timestamp)
          n254 = local read "TestTime"() -> (w731:dbl)
          n255 = To Double Precision Float(number=w732) -> (double precision float=w730:dbl)
          n256 = shared-variable "My Computer\\michelle_library.lvlib\\InitiatedLag"() -> (w729:dbl)  [unwired: 1 in, 1 out]
          n257 = Subtract(x=w730, y=w731) -> (x-y=w727:dbl)
          n258 = Subtract(x=w727, y=w729) -> (x-y=→"Lag2":dbl)
        }
        frame #2 {
          n259 = local read "TestTime"() -> (w733:dbl)
          n260 = local read "Lag2"() -> (w734:dbl)
          n261 = Add(x=w733, y=w734) -> (x+y=w735:dbl)
          n262 = local write "TestTime"(w735) -> ()
        }
        frame #3 {
          n263 = shared-variable "My Computer\\michelle_library.lvlib\\Timings"() -> (→"Timings":dbl[])  [unwired: 1 in, 1 out]
          n264 = shared-variable "My Computer\\michelle_library.lvlib\\Stim_ID"() -> (→"Stim_ID":dbl[])  [unwired: 1 in, 1 out]
          n265 = Wait (ms)(milliseconds to wait=u32 10) -> ()  [unwired: 1 out]
          n266 = shared-variable "My Computer\\michelle_library.lvlib\\Reward_mat"() -> (→"Reward_mat":dbl[])  [unwired: 1 in, 1 out]
          n267 = shared-variable "My Computer\\michelle_library.lvlib\\Num_trials"() -> (w739:u32)  [unwired: 1 in, 1 out]
          n268 = Initialize Array(0.0 ("element"), w739) -> (→"Rewarded trials":dbl[])
        }
        frame #4 {
          n269 = while {
            shift-right: [w855] -> _
            shift-left: _ -> [w853]
            shift-right: [w851] -> _
            shift-left: _ -> [w850]
            shift-right: [w845] -> _
            shift-left: _ -> [w843]
            stop <- w856 stop-if-true
            n270 = local read "ConsumptionGo"() -> (w845:bool)
            n271 = shared-variable "My Computer\\michelle_library.lvlib\\Display"() -> (w851:bool)  [unwired: 1 in, 1 out]
            n272 = local read "Time_out"() -> (w855:bool)
            n273 = Wait (ms)(milliseconds to wait=u32 10) -> ()  [unwired: 1 out]
            n274 = Not(x=w855) -> (.not. x?=w854:bool)
            n275 = Not(x=w851) -> (.not. x?=w849:bool)
            n276 = Not(x=w845) -> (.not. x?=w846:bool)
            n277 = And(x=w854, y=w853) -> (x .and. y?=w848:bool)
            n278 = And(x=w850, y=w849) -> (x .and. y?=w844:bool)
            n279 = local read "Time_out"() -> (w852:bool)
            n280 = And(x=w843, y=w846) -> (x .and. y?=w842:bool)
            n281 = Or(x=w848, y=w844) -> (x .or. y?=w841:bool)
            n282 = Or(x=w841, y=w842) -> (x .or. y?=w840:bool)
            n283 = case shown="True" w840 {
              tunnel: w852 -> [w857 _]
              frame False {
                n284 = case shown="False" w857 {
                  frame False {
                    n285 = local read "ISI start time"() -> (w860:dbl)
                    n286 = local read "Time"() -> (w859:dbl)
                    n287 = Subtract(x=w859, y=w860) -> (x-y=w858:dbl)
                    n288 = shared-variable "My Computer\\michelle_library.lvlib\\ISI"(w858) -> ()  [unwired: 1 in, 1 out]
                    n289 = local write "ISI"(w858) -> ()
                  }
                  frame True {
                    n290 = local read "Time"() -> (w865:dbl)
                    n291 = Subtract(x=w865, y=0.11) -> (x-y=w862:dbl)
                    n292 = local write "ISI start time"(w862) -> ()
                    n293 = local read "Time"() -> (w863:dbl)
                    n294 = Subtract(x=w863, y=w862) -> (x-y=w861:dbl)
                    n295 = shared-variable "My Computer\\michelle_library.lvlib\\ISI"(w861) -> ()  [unwired: 1 in, 1 out]
                    n296 = local write "ISI"(w861) -> ()
                  }
                }
              }
              frame True {
                n297 = local read "Time"() -> (w870:dbl)
                n298 = Subtract(x=w870, y=0.11) -> (x-y=w867:dbl)
                "ISI start time" <- w867
                n299 = local read "Time"() -> (w868:dbl)
                n300 = Subtract(x=w868, y=w867) -> (x-y=w866:dbl)
                "ISI" <- w866
                n301 = shared-variable "My Computer\\michelle_library.lvlib\\ISI"(w866) -> ()  [unwired: 1 in, 1 out]
              }
            }
            n302 = local read "Stop"() -> (w856:bool)
          }
          n303 = while {
            stop <- w745 stop-if-true
            n304 = local read "Active Trial"() -> (w744:bool)
            n305 = case shown="True" w744 {
              frame False {
              }
              frame True {
                n306 = local write "Time_out"(FALSE) -> ()
                n307 = shared-variable "My Computer\\michelle_library.lvlib\\Timeout"(FALSE) -> ()  [unwired: 1 in, 1 out]
              }
            }
            n308 = Wait (ms)(milliseconds to wait=5) -> ()  [unwired: 1 out]
            n309 = shared-variable "My Computer\\michelle_library.lvlib\\Stop"() -> (w745:bool)  [unwired: 1 in, 1 out]
          }
          n310 = while {
            stop <- w766 stop-if-true
            n311 = shared-variable "My Computer\\michelle_library.lvlib\\Trial"() -> (w756:u32)  [unwired: 1 in, 1 out]
            n312 = Wait (ms)(milliseconds to wait=u32 10) -> ()  [unwired: 1 out]
            n313 = local read "Timings"() -> (w758:dbl[])
            n314 = local read "Time since lick"() -> (w765:dbl)
            n315 = Decrement(x=w756) -> (x-1=w755:u32)
            n316 = Index Array(array=w758, index=w755) -> (element=w757:dbl)
            n317 = Less?(x=w765, y=w757) -> (x < y?=w764:bool)
            n318 = shared-variable "My Computer\\michelle_library.lvlib\\Display"() -> (w761:bool)  [unwired: 1 in, 1 out]
            n319 = local read "ConsumptionGo"() -> (w753:bool)
            n320 = local read "Lick"() -> (w763:bool)
            n321 = And(x=w763, y=w764) -> (x .and. y?=w759:bool)
            n322 = Not(x=w761) -> (.not. x?=w760:bool)
            n323 = local read "Active Trial"() -> (w748:bool)
            n324 = And(x=w760, y=w759) -> (x .and. y?=w752:bool)
            n325 = Not(x=w753) -> (.not. x?=w754:bool)
            n326 = And(x=w752, y=w754) -> (x .and. y?=w750:bool)
            n327 = Not(x=w748) -> (.not. x?=w751:bool)
            n328 = And(x=w750, y=w751) -> (x .and. y?=w749:bool)
            n329 = case shown="True" w749 {
              frame False {
              }
              frame True {
                n330 = flat-sequence {
                  frame #0 {
                    w767 = TRUE
                    n331 = local read "TimeOutDuration"() -> (w768:i32)
                    n332 = xnode "DisplayOn 3"("C/DIO3 (DIO3)"=w767) -> ()  [unwired: 1 in, 1 out]
                    n333 = shared-variable "My Computer\\michelle_library.lvlib\\Timeout"(w767) -> ()  [unwired: 1 in, 1 out]
                    n334 = Wait (ms)(milliseconds to wait=w768) -> ()  [unwired: 1 out]
                    "Time_out" <- w767
                  }
                  frame #1 {
                    w804 = FALSE ("Timeout")
                    n335 = xnode "DisplayOn 4"("C/DIO3 (DIO3)"=w804) -> ()  [unwired: 1 in, 1 out]
                    n336 = local write "Time_out"(w804) -> ()
                    n337 = shared-variable "My Computer\\michelle_library.lvlib\\Timeout"(w804) -> ()  [unwired: 1 in, 1 out]
                  }
                }
              }
            }
            n338 = local read "Stop"() -> (w766:bool)
          }
          n339 = while {
            shift-right: [w917] -> _
            shift-left: _ -> [w916]
            shift-right: [w909] -> _
            shift-left: _ -> [w910]
            stop <- w919 stop-if-true
            n340 = local read "Active Trial"() -> (w914:bool)
            n341 = Wait (ms)(milliseconds to wait=u32 10) -> ()  [unwired: 1 out]
            n342 = local read "Lick"() -> (w915:bool)
            n343 = And(x=w914, y=w915) -> (x .and. y?=w913:bool)
            n344 = Or(x="Give reward", y=w913) -> (x .or. y?=w912:bool)
            n345 = case shown="True" w912 {
              tunnel: [w921 w928] -> w917
              tunnel: w916 -> [w921 w927]
              tunnel: w910 -> [w920 w925]
              tunnel: [w920 w924] -> w909
              frame False {
              }
              frame True {
                n346 = flat-sequence {
                  tunnel: w925 -> [w934]
                  tunnel: [w931] -> w922
                  tunnel: [w990] -> w923
                  tunnel: w922 -> [w988]
                  tunnel: [w1034] -> w924
                  tunnel: w923 -> [w1034]
                  frame #0 {
                    w949 = TRUE ("C/DIO0 (DIO0)")
                    n347 = Get Date/Time In Seconds() -> (seconds since 1Jan1904=w938:timestamp)
                    n348 = local write "Time_out"(FALSE) -> ()
                    n349 = shared-variable "My Computer\\michelle_library.lvlib\\Timeout"(FALSE) -> ()  [unwired: 1 in, 1 out]
                    n350 = local write "GoAhead"(FALSE) -> ()
                    n351 = Wait (ms)(milliseconds to wait=u32 100) -> ()  [unwired: 1 out]
                    n352 = local read "TestTime"() -> (w932:dbl)
                    n353 = shared-variable "My Computer\\michelle_library.lvlib\\Trial"() -> (w948:u32)  [unwired: 1 in, 1 out]
                    n354 = shared-variable "My Computer\\michelle_library.lvlib\\GlobalReward"() -> (w940:dbl)  [unwired: 1 in, 1 out]
                    n355 = To Double Precision Float(number=w938) -> (double precision float=w937:dbl)
                    n356 = shared-variable "My Computer\\michelle_library.lvlib\\GlobalTime"() -> (w930:dbl)  [unwired: 1 in, 1 out]
                    n357 = local read "Rewarded trials"() -> (w946:dbl[])
                    n358 = Subtract(x=w937, y=w932) -> (x-y=w936:dbl)
                    n359 = xnode "Reward 3"("C/DIO0 (DIO0)"=w949) -> ()  [unwired: 1 in, 1 out]
                    n360 = Decrement(x=w948) -> (x-1=w947:u32)
                    n361 = shared-variable "My Computer\\michelle_library.lvlib\\Frame_clock"() -> (w929:u32)  [unwired: 1 in, 1 out]
                    n362 = Increment(x=w940) -> (x+1=w939:dbl)
                    n363 = Replace Array Subset(array=w946, new element=1.0 ("new element/subarray"), index=w947) -> (w944:dbl[])
                    n364 = Build Array(551, w936, w930, w929) -> (w935:T1)
                    n365 = local write "Rewarded trials"(w944) -> ()
                    n366 = shared-variable "My Computer\\michelle_library.lvlib\\GlobalReward"(w939) -> ()  [unwired: 1 in, 1 out]
                    n367 = Build Array (concatenate) ("Build Matrix")(w934, w935) -> (w931:T1)
                    n368 = local write "RewTS"(w931) -> ()
                    "Reward" <- w949
                    "Watch_Display" <- w949
                  }
                  frame #1 {
                    w998 = FALSE ("C/DIO0 (DIO0)")
                    n369 = Get Date/Time In Seconds() -> (seconds since 1Jan1904=w995:timestamp)
                    n370 = local read "TestTime"() -> (w989:dbl)
                    n371 = local write "Give reward"(FALSE ("Give reward")) -> ()
                    n372 = Wait (ms)(milliseconds to wait=u32 20) -> ()  [unwired: 1 out]
                    n373 = shared-variable "My Computer\\michelle_library.lvlib\\GlobalTime"() -> (w987:dbl)  [unwired: 1 in, 1 out]
                    n374 = To Double Precision Float(number=w995) -> (double precision float=w994:dbl)
                    n375 = xnode "Reward 4"("C/DIO0 (DIO0)"=w998) -> ()  [unwired: 1 in, 1 out]
                    n376 = local write "Reward"(w998) -> ()
                    n377 = Subtract(x=w994, y=w989) -> (x-y=w993:dbl)
                    n378 = shared-variable "My Computer\\michelle_library.lvlib\\Frame_clock"() -> (w986:u32)  [unwired: 1 in, 1 out]
                    n379 = Build Array(552, w993, w987, w986) -> (w991:T1)
                    n380 = Build Array (concatenate) ("Build Matrix")(w988, w991) -> (w990:T1)
                    n381 = local write "RewTS"(w990) -> ()
                  }
                  frame #2 {
                    n382 = Wait (ms)(milliseconds to wait=u32 50) -> ()  [unwired: 1 out]
                  }
                }
                n383 = Increment(x=w927) -> (x+1=w928:u16)
                "Rewards" <- w928
                n384 = local write "Active Trial"(FALSE ("Active Trial")) -> ()
              }
            }
            n385 = local read "Stop"() -> (w919:bool)
          }
          n386 = while {
            stop <- w884 stop-if-true
            n387 = shared-variable "My Computer\\michelle_library.lvlib\\Trial"() -> (w880:u32)  [unwired: 1 in, 1 out]
            n388 = shared-variable "My Computer\\michelle_library.lvlib\\Trial"() -> (w876:u32)  [unwired: 1 in, 1 out]
            n389 = Wait (ms)(milliseconds to wait=u32 10) -> ()  [unwired: 1 out]
            n390 = local read "Rewarded trials"() -> (w877:dbl[])
            n391 = local read "Reward_mat"() -> (w879:dbl[])
            n392 = Decrement(x=w880) -> (x-1=w881:u32)
            n393 = Decrement(x=w876) -> (x-1=w875:u32)
            n394 = Index Array(array=w879, index=w881) -> (element=w882:dbl)
            n395 = Index Array(array=w877, index=w875) -> (element=w874:dbl)
            n396 = Equal To 0?(x=w874) -> (x = 0?=w873:bool)
            n397 = Equal?(x=w882, y=1.0) -> (x = y?=w872:bool)
            n398 = And(x=w872, y=w873) -> (x .and. y?=w871:bool)
            n399 = case shown="True" w871 {
              frame False {
                n400 = local write "Active Trial"(FALSE ("Active_trial")) -> ()
              }
              frame True {
                n401 = shared-variable "My Computer\\michelle_library.lvlib\\Trial"() -> (w887:u32)  [unwired: 1 in, 1 out]
                n402 = local read "Stim_ID"() -> (w889:dbl[])
                n403 = Decrement(x=w887) -> (x-1=w888:u32)
                n404 = Index Array(array=w889, index=w888) -> (element=w886:dbl)
                n405 = case shown="1, Default" w886 {
                  frame 1, Default {
                    n406 = shared-variable "My Computer\\michelle_library.lvlib\\ISI_Time"() -> (w895:dbl)  [unwired: 1 in, 1 out]
                    n407 = local read "ActiveTime"() -> (w890:dbl)
                    n408 = Less?(x=w895, y=w890) -> (x < y?=w893:bool)
                    n409 = Greater?(x=w895, y=0.1) -> (0:w892:bool)
                    n410 = And(x=w893, y=w892) -> (x .and. y?=w891:bool)
                    n411 = case shown="True" w891 {
                      frame False {
                        n412 = local write "Active Trial"(FALSE ("Active Trial")) -> ()
                      }
                      frame True {
                        n413 = local read "Time"() -> (w899:dbl)
                        n414 = local write "Active Trial"(TRUE ("Active Trial")) -> ()
                        n415 = Add(x=w899, y=-0.11) -> (x+y=w897:dbl)
                        n416 = local write "Time of last lick"(w897) -> ()
                      }
                    }
                  }
                  frame 2 {
                    n417 = shared-variable "My Computer\\michelle_library.lvlib\\ISI_Time"() -> (w905:dbl)  [unwired: 1 in, 1 out]
                    n418 = local read "ActiveTime"() -> (w901:dbl)
                    n419 = Less?(x=w905, y=w901) -> (x < y?=w903:bool)
                    n420 = Greater?(x=w905, y=0.1) -> (0:w904:bool)
                    n421 = And(x=w904, y=w903) -> (x .and. y?=w902:bool)
                    n422 = case shown="True" w902 {
                      frame False {
                        n423 = local write "Active Trial"(FALSE ("Active Trial")) -> ()
                      }
                      frame True {
                        "Active Trial" <- TRUE ("Active Trial")
                      }
                    }
                  }
                }
              }
            }
            n424 = local read "Stop"() -> (w884:bool)
          }
        }
      }
      n425 = while {
        shift-right: [w346] -> _
        shift-left: _ -> [w341]
        stop <- w345 stop-if-true
        n426 = xnode "PhotoDiode"() -> ("C/AI0 (AI0)"=w342:dbl)  [unwired: 1 in, 1 out]
        "Light" <- w342
        n427 = Wait (ms)(milliseconds to wait=u32 10) -> ()  [unwired: 1 out]
        n428 = Build Array (concatenate)(w341, w342) -> (w346:dbl[])
        "Lightplot" <- w346
        "LightArray" <- w346
        n429 = Greater?(x=w342, y=0.5) -> (0:→"LightOn":bool)
        n430 = local read "Stop"() -> (w345:bool)
      }
      n431 = flat-sequence {
        frame #0 {
          n432 = xnode "Encoder 4"("Reset Counter"=TRUE) -> ()  [unwired: 1 in, 4 out]
        }
        frame #1 {
          n433 = while {
            shift-right: [w438] -> _
            shift-left: _ -> [w439]
            stop <- w443 stop-if-true
            n434 = local read "GetVidFrame"() -> (w433:i32)
            n435 = local read "VidFrameClock"() -> (w437:i32)
            n436 = Equal?(x=w437, y=1) -> (x = y?=w436:bool)
            n437 = Equal?(x=w433, y=1) -> (x = y?=w432:bool)
            n438 = And(x=w436, y=w432) -> (x .and. y?=w435:bool)
            n439 = case shown="True" w435 {
              tunnel: w439 -> [w447 w450]
              tunnel: [w447 w449] -> w438
              frame False {
              }
              frame True {
                n440 = local read "TestTime"() -> (w456:dbl)
                n441 = shared-variable "My Computer\\michelle_library.lvlib\\GlobalTime"() -> (w453:dbl)  [unwired: 1 in, 1 out]
                n442 = Get Date/Time In Seconds() -> (seconds since 1Jan1904=w458:timestamp)
                n443 = shared-variable "My Computer\\michelle_library.lvlib\\Frame_clock"() -> (w454:u32)  [unwired: 1 in, 1 out]
                n444 = To Double Precision Float(number=w458) -> (double precision float=w457:dbl)
                n445 = Subtract(x=w457, y=w456) -> (x-y=w455:dbl)
                n446 = Build Array(881, w455, w453, w454) -> (w452:T1)
                n447 = Build Array (concatenate) ("Build Matrix")(w450, w452) -> (w449:T1)
                n448 = local write "GetVidFrame"(0) -> ()
                n449 = local write "VidTS"(w449) -> ()
              }
            }
            n450 = xnode "Encoder 3"() -> ("Counter Value"=w445:i32)  [unwired: 2 in, 3 out]
            n451 = Multiply(x=w445, y=-1) -> (x*y=w442:i32)
            "VidFrameClock" <- w442
            n452 = Equal?(x=w442, y=720000) -> (x = y?=w443:bool)
            n453 = shared-variable "My Computer\\michelle_library.lvlib\\VidFrameClock1"(w442) -> ()  [unwired: 1 in, 1 out]
            n454 = local write "Stop"(w443) -> ()
            n455 = Wait (ms)(milliseconds to wait=u32 1) -> ()  [unwired: 1 out]
          }
        }
        frame #2 {
          n456 = local read "Stop"() -> (w505:bool)
          n457 = shared-variable "My Computer\\michelle_library.lvlib\\Stop"(w505) -> ()  [unwired: 1 in, 1 out]
        }
      }
    }
  }
